vi "WFDC Check CC Errors.vi"(0 "Fit Result":dbl[](array[numeric]), 5 "CC Image":dbl[][](array[numeric]), 7 "Contrast Limit":dbl, 9 "Roundness Limit":dbl, 11 "Error In":errorcluster) -> (15 "Error Out":errorcluster)   [LabVIEW 2020]
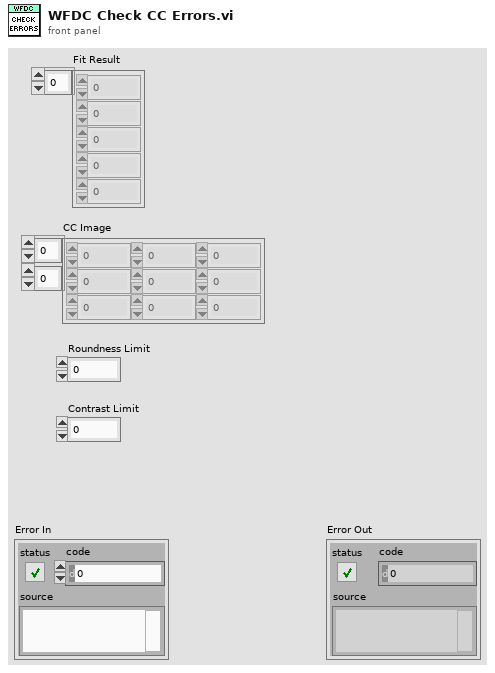
[diagram p1: front panel]
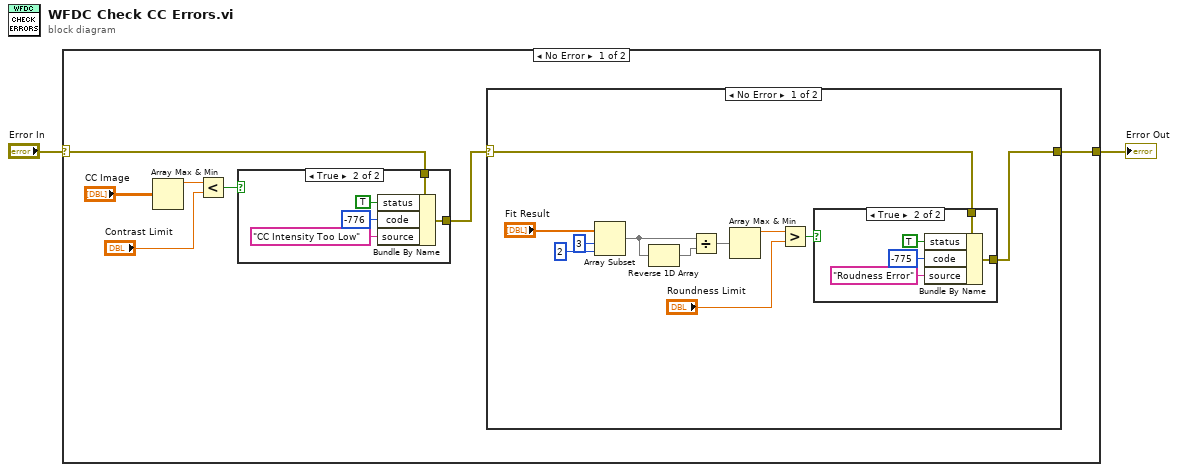
[diagram p0: block diagram]
diagram:
  n1 = case shown="No Error" "Error In" {
    selector: "Error In" -> [w5 w34]
    tunnel: [w3 w34] -> w1
    frame No Error {
      n2 = Array Max & Min(array="CC Image") -> (max value=w9:dbl)  [unwired: 3 out]
      n3 = Less?(x=w9, y="Contrast Limit") -> (x < y?=w8:bool)
      n4 = case shown="True" w8 {
        tunnel: w5 -> [w10 w12]
        tunnel: [w10 w11] -> w4
        frame False {
        }
        frame True {
          n5 = Bundle By Name(cluster=w12, "status"=TRUE, "code"=-776, "source"="CC Intensity Too Low") -> (w11:errorcluster)
        }
      }
      n6 = case shown="No Error" w4 {
        selector: w4 -> [w17 w33]
        tunnel: [w16 w33] -> w3
        frame No Error {
          n7 = Array Subset(array="Fit Result", index=3, length=2) -> (w22:dbl[])
          n8 = Reverse 1D Array(array=w22) -> (reversed array=w23:dbl[])
          n9 = Divide(x=w22, y=w23) -> (x/y=w24:dbl[])
          n10 = Array Max & Min(array=w24) -> (max value=w21:dbl)  [unwired: 3 out]
          n11 = Greater?(x=w21, y="Roundness Limit") -> (0:w20:bool)
          n12 = case shown="True" w20 {
            tunnel: w17 -> [w27 w29]
            tunnel: [w27 w28] -> w16
            frame False {
            }
            frame True {
              n13 = Bundle By Name(cluster=w29, "status"=TRUE, "code"=-775, "source"="Roudness Error") -> (w28:errorcluster)
            }
          }
        }
        frame Error {
        }
      }
    }
    frame Error {
    }
  }
  "Error Out" <- w1
